vi "SYST_SHOR_TITL.vi"(0 "VISA IN":refnum<visa-resource-name>, 1 "Macro":string, 5 "error in":errorcluster, 7 "Number":i32) -> (14 "VISA Out":refnum<visa-resource-name>, 19 "error out":errorcluster)   [LabVIEW 2018, in "PNA-X.lvlib"]
doc: "SYSTem:SHORtcut<n>:TITLe<string> \n1883\n\n(Read-Write) Reads and writes the name of the specified macro. \nParameters \n<n> Numeric. Number of the macro that is stored in the PNA. \nTo find the number of a macro, either open the Macro Setup dialog and count \nthe line number of the desired macro, or query the titles of all 12 macros for the \ndesired macro title. \n<string> The name to be assigned to the macro. \nExamples SYST:SHOR1:TITL \"Guided 4-Port Cal\" \nQuery Syntax SYSTem:SHORtcut<n>:TITLe? \nDefault Not Applicable"
uses:
  PNA-X.lvlib
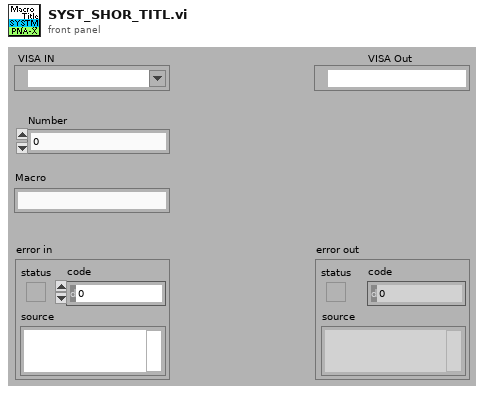
[diagram p1: front panel]
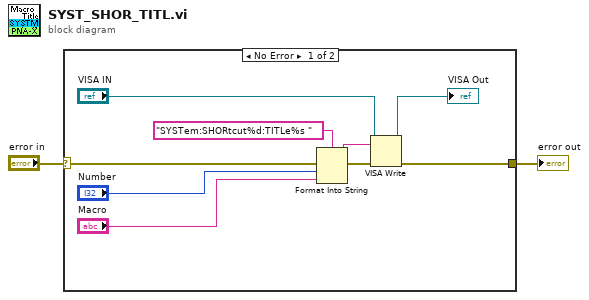
[diagram p0: block diagram]
diagram:
  n1 = case shown="No Error" "error in" {
    selector: "error in" -> [w11 w12]
    tunnel: [w6 w12] -> w1
    frame No Error {
      n2 = Format Into String(format string="SYSTem:SHORtcut%d:TITLe%s " ("Cmdline"), error in=w11, "Number", "Macro") -> (resulting string=w9:string, error out=w10:errorcluster)  [unwired: 1 in]
      n3 = VISA Write(VISA resource name="VISA IN", write buffer=w9, error in (no error)=w10) -> (VISA resource name out=→"VISA Out":refnum<visa-resource-name>, error out=w6:errorcluster)  [unwired: 1 out]
    }
    frame Error {
    }
  }
  "error out" <- w1
